vi "Configure Alarms.vi"(8 "error in (no error)":errorcluster, 11 "CryoCoolerAVC in":refnum<class "CryoCoolerAVC.lvclass">) -> (0 "error out":errorcluster, 3 "CryoCoolerAVC out":refnum<class "CryoCoolerAVC.lvclass">)   [LabVIEW 2022 SP3, in "CryoCoolerAVC.lvclass"]
uses:
  CryoCoolerAVC.lvclass
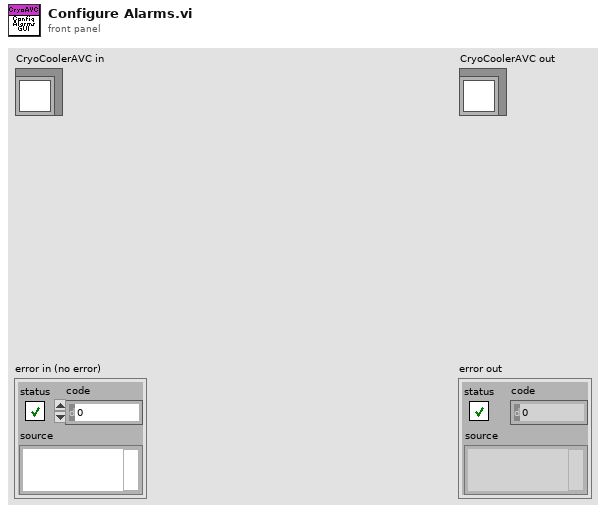
[diagram p1: front panel]
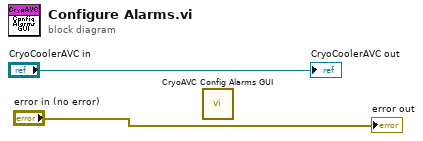
[diagram p0: block diagram]
diagram:
  n1 = call "CryoAVC Config Alarms GUI.vi"() -> ()  [unwired: 11 in, 1 out]
  "error out" <- "error in (no error)"
  "CryoCoolerAVC out" <- "CryoCoolerAVC in"
